vi "Interpolate Standard Data.vi"(0 "Standard Data":T1[](array[typedef]), 5 "Cal Frequencies":dbl[](array[numeric]), 11 "error in (no error)":errorcluster) -> (4 "Interpolated Standard Data":T1[](array[typedef]), 15 "error out":errorcluster)   [LabVIEW 2023, in "RFFixtureCharact.Public.lvlib" / "Vector Abstract Path.lvclass"]
uses:
  Vector Abstract Path.lvclass
  Instruments/Cal Standard/Type Definitions/One-Port Charact Data.ctl
  Instruments/Cal Standard/Type Definitions/Standard Type.ctl
  Vector Abstract Path.lvclass/Vector Abstract Path.ctl
  Dependencies/HFNetworkAnalysis/NI_HFNetworkAnalysis.lvlib
  Instruments/RFFixtureCharact.Instruments.lvlib
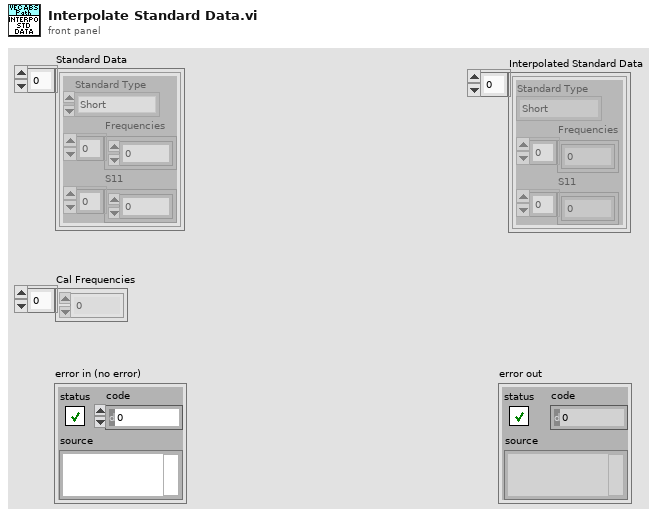
[diagram p1: front panel]
types:
  T1 = typedef "RFFixtureCharact.Instruments.lvlib/One-Port Charact Data.ctl" = cluster{"Standard Type":T2, "Frequencies":dbl[], "S11":cdb[]}
  T2 = typedef "RFFixtureCharact.Instruments.lvlib/Standard Type.ctl" = enum16{"Short", "Open", "Load", "PowerMeter", "None"}
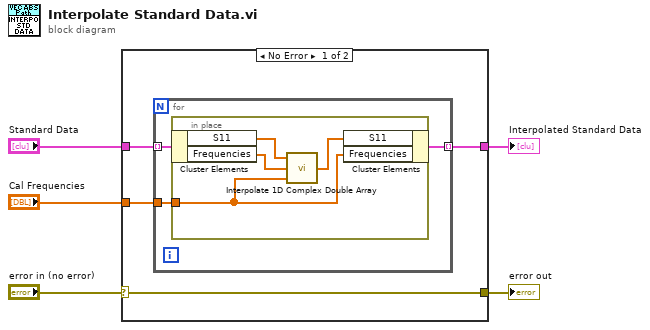
[diagram p0: block diagram]
diagram:
  n1 = case shown="No Error" "error in (no error)" {
    selector: "error in (no error)" -> [w9 w18]
    tunnel: [w9 w18] -> w4
    tunnel: "Cal Frequencies" -> [w8 _]
    tunnel: "Standard Data" -> [w7 w17]
    tunnel: [w6 w17] -> w1
    frame No Error {
      n2 = for {
        tunnel: w8 -> [w12]
        tunnel: w7 -> [w11] mode=indexing
        tunnel: [w10] -> w6 mode=indexing
        n3 = in-place {
          in-place-border: w12 -> [w13]
          n4 = in-place-cluster #1(w11) -> ("S11"=w15:cdb[], "Frequencies"=w16:dbl[])
          n5 = call "Interpolate 1D Complex Double Array.vi"("xi"=w13, "X"=w16, "Y"=w15) -> ("yi"=w14:cdb[])
          n6 = in-place-cluster #1("S11"=w14, "Frequencies"=w13) -> (w10:T1)
        }
      }
    }
    frame Error {
    }
  }
  "error out" <- w4
  "Interpolated Standard Data" <- w1
